vi "Move Bounding Window.vi"(2 "load data":T1={"max address"=0.0, "Memory"="Digital Pattern Gen Memory 0"}, 5 "State Data":T2) -> (0 "Memory Lookup":fxp<+,10,10>, 1 "State Data Out":T2)   [LabVIEW 2015, in "Engine Simulation Toolkit.lvlib" / "Directional Speed.lvlib"]
uses:
  Directional Speed.lvlib
  State Data.ctl
  Settings.ctl
  State.ctl
  Load Data.ctl
  Engine Simulation Toolkit.lvlib
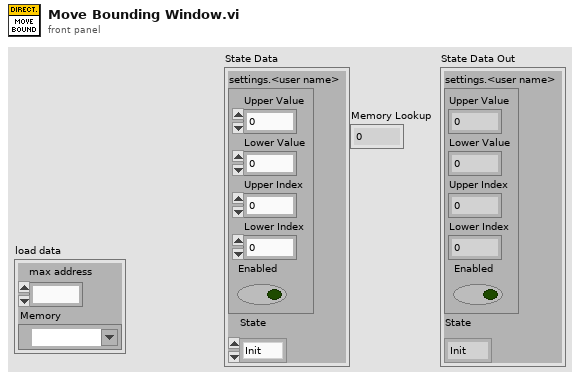
[diagram p1: front panel]
types:
  T1 = typedef "Engine Simulation Toolkit.lvlib/Directional Speed.lvlib/Load Data.ctl" = cluster{"max address":fxp<+,10,10>, "Memory":refnum<k21>}
  T2 = typedef "Engine Simulation Toolkit.lvlib/Directional Speed.lvlib/State Data.ctl" = cluster{"settings.<user name>":T3, "State":T4}
  T3 = typedef "Engine Simulation Toolkit.lvlib/Directional Speed.lvlib/Settings.ctl" = cluster{"Upper Value":u16, "Lower Value":u16, "Upper Index":fxp<+,10,10>, "Lower Index":fxp<+,10,10>, "Enabled":bool}
  T4 = typedef "Engine Simulation Toolkit.lvlib/Directional Speed.lvlib/State.ctl" = enum8{"Init", "Detect", "Positive Move td", "Negative Move td", "tf", "tr"}
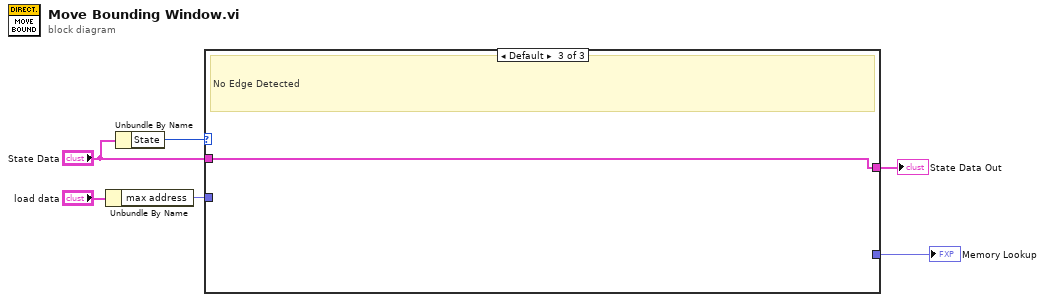
[diagram p0: block diagram]
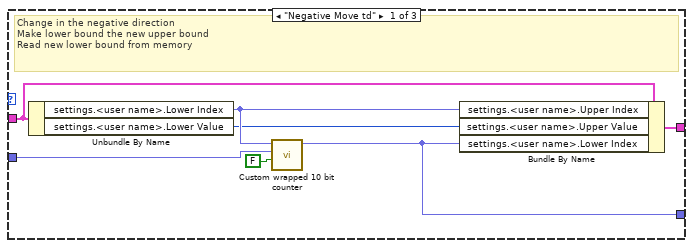
[diagram p2: hidden frame]
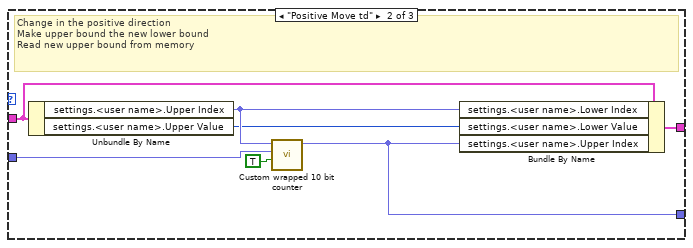
[diagram p3: hidden frame]
diagram:
  n1 = Unbundle By Name("load data") -> ("max address"=w5:fxp<+,10,10>)
  n2 = Unbundle By Name("State Data") -> ("State"=w4:T4)
  n3 = case shown="Default" w4 {
    tunnel: w5 -> [w12 w19 _]
    tunnel: "State Data" -> [w11 w18 w21]
    tunnel: [w10 w16 w21] -> w2
    tunnel: [w7 w14 _] -> w1
    frame "Negative Move td" {
      # "Change in the negative direction\nMake lower bound the new upper bound\nRead new lower bound from memory"
      n4 = Unbundle By Name(w11) -> ("settings.<user name>.Lower Index"=w9:fxp<+,10,10>, "settings.<user name>.Lower Value"=w8:u16)
      n5 = call "Custom wrapped 10 bit counter.vi"("increment or decrement (decrement)"=FALSE, "max value"=w12, "value"=w9) -> ("new value"=w7:fxp<+,10,10>)  [unwired: 7 in, 1 out]
      n6 = Bundle By Name(cluster=w11, "settings.<user name>.Upper Index"=w9, "settings.<user name>.Upper Value"=w8, "settings.<user name>.Lower Index"=w7) -> (w10:T2)
    }
    frame "Positive Move td" {
      # "Change in the positive direction\nMake upper bound the new lower bound\nRead new upper bound from memory"
      n7 = Unbundle By Name(w18) -> ("settings.<user name>.Upper Index"=w17:fxp<+,10,10>, "settings.<user name>.Upper Value"=w15:u16)
      n8 = call "Custom wrapped 10 bit counter.vi"("increment or decrement (decrement)"=TRUE, "max value"=w19, "value"=w17) -> ("new value"=w14:fxp<+,10,10>)  [unwired: 7 in, 1 out]
      n9 = Bundle By Name(cluster=w18, "settings.<user name>.Lower Index"=w17, "settings.<user name>.Lower Value"=w15, "settings.<user name>.Upper Index"=w14) -> (w16:T2)
    }
    frame Default {
      # "No Edge Detected"
    }
  }
  "State Data Out" <- w2
  "Memory Lookup" <- w1
